vi "subHamamatsu_Snapshot.vi"(7 "Frames to average (1)":i32=1, 8 "Error in":errorcluster, 11 "Value":u32) -> (0 "Error out":errorcluster, 2 "Image":u16[][](graph), 3 "Handle out":u32)   [LabVIEW 2015]
panel:
  # "Take a snapshot and average"
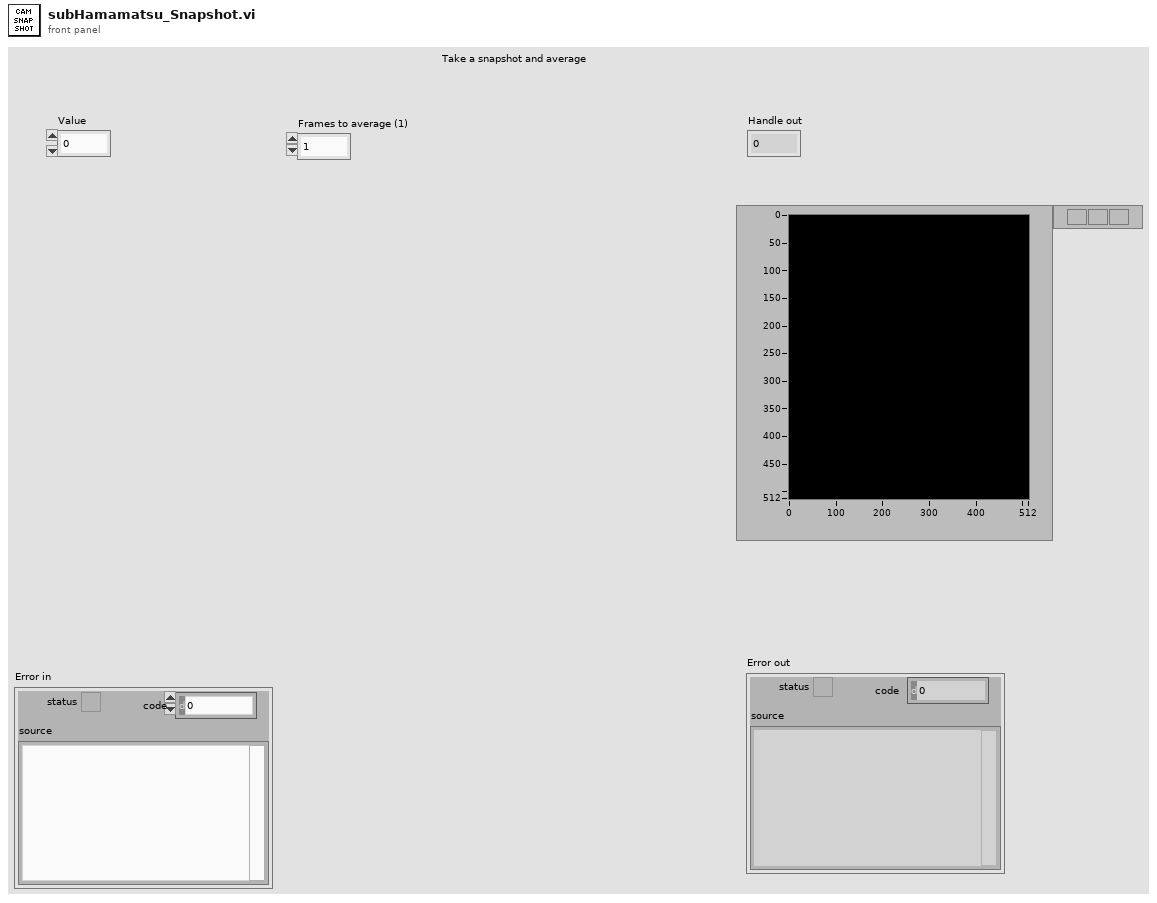
[diagram p1: front panel]
types:
  T1 = cluster{"Value":i32, "Minimum":i32, "Maximum":i32, "Increment":i32}
  T2 = cluster{"width":u32, "height":u32, "datatype":u32}
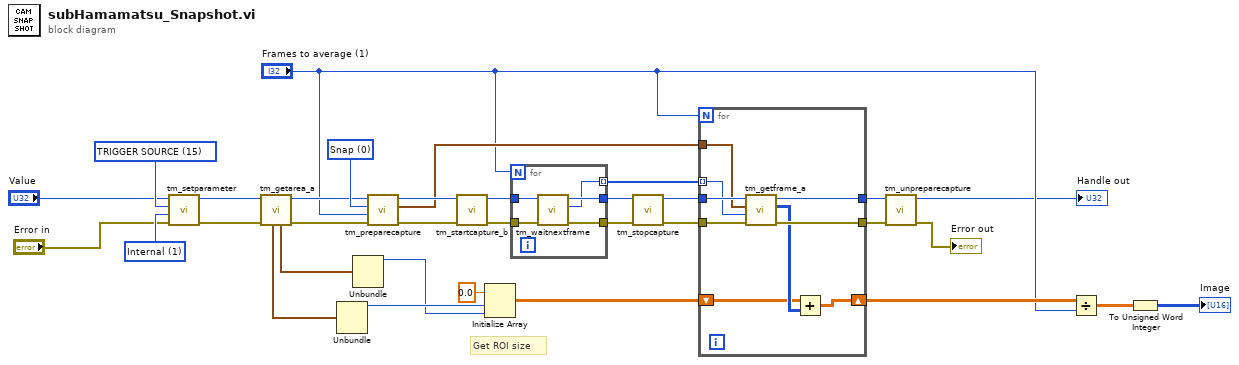
[diagram p0: block diagram]
diagram:
  w32 = 1 items=["Internal"=1, "External"=2, "Software"=3] ("Trigger Source")
  w33 = 15 items=["BINNING"=1, "BITS PER CHANNEL"=2, "ACTIVE VIEW INDEX"=3, "CCD MODE"=4, "SENSOR MODE"=5, "READOUT MODE"=6, "EXPOSURE TIME"=7, "CONTRAST GAIN"=8, "CONTRAST OFFSET"=9, "LIGHT MODE"=10, "SENSITIVITY"=11, "WHITE BALANCE"=12, "PHOTON IMAGING MODE"=13, "HIGH DYNAMIC RANGE MODE"=14, "TRIGGER SOURCE"=15, "TRIGGER ACTIVE"=16, "TRIGGER MODE"=17, "TRIGGER POLARITY"=18, "TRIGGER GLOBAL EXPOSURE"=19, "FIRST TRIGGER BEHAVIOR"=20, "TRIGGER TIMES"=21, "OUTPUT TRIGGER POLARITY"=22, "OUTPUT TRIGGER DELAY"=23, "OUTPUT TRIGGER PERIOD"=24, "TEMPERATURE"=25, "TEMPERATURE TARGET"=26, "SENSOR COOLER FAN"=27, "MECHANICAL SHUTTER"=28, "BACK FOCUS POSITION"=29, "FRAMEBUNDLE MODE"=30, "FRAMEBUNDLE NUMBER"=31, "LINEBUNDLE HEIGHT"=32, "TRIGGER CONNECTOR"=33, "IMAGE PIXEL TYPE"=34] ("Parameter")
  w31 = 0 items=["Snap", "Sequence"] ("Capture mode")
  # "Get ROI size"
  n1 = call "tm_setparameter.vi"("error in (no error)"="Error in", "Value in"=w32, "Parameter"=w33, "Handle in"="Value") -> ("error out"=w3:errorcluster, "Handle out"=w4:u32)  [unwired: 6 in]
  n2 = call "tm_getarea_a.vi"("error in (no error)"=w3, "Handle in"=w4) -> ("error out"=w6:errorcluster, "Handle out"=w7:u32, "H Width"=w11:T1, "V Width"=w12:T1)  [unwired: 4 in, 2 out]
  n3 = Unbundle(w12) -> ("Value"=w10:i32)  [unwired: 3 out]
  n4 = Unbundle(w11) -> ("Value"=w9:i32)  [unwired: 3 out]
  n5 = call "tm_preparecapture.vi"("error in (no error)"=w6, "Frames"="Frames to average (1)", "Capture mode"=w31, "Handle in"=w7) -> ("error out"=w22:errorcluster, "Buffer"=w20:T2, "Handle out"=w21:u32)  [unwired: 4 in, 1 out]
  n6 = call "tm_startcapture_b.vi"("error in (no error)"=w22, "Handle in"=w21) -> ("error out"=w25:errorcluster, "Handle out"=w24:u32)  [unwired: 8 in]
  n7 = Initialize Array(0.0 ("element"), w10, w9) -> (w8:dbl[][])
  n8 = for {
    N: "Frames to average (1)" -> [_]
    tunnel: w24 -> [w38]
    tunnel: w25 -> [w37]
    tunnel: [w36] -> w27
    tunnel: [w35] -> w26
    tunnel: [w34] -> w28 mode=indexing
    n9 = call "tm_waitnextframe.vi"("error in (no error)"=w37, "Handle in"=w38) -> ("error out"=w36:errorcluster, "Frame Index"=w34:i32, "Handle out"=w35:u32)  [unwired: 6 in, 1 out]
  }
  n10 = call "tm_stopcapture.vi"("error in (no error)"=w27, "Handle in"=w26) -> ("error out"=w14:errorcluster, "Handle out"=w15:u32)  [unwired: 8 in]
  n11 = for {
    N: "Frames to average (1)" -> [_]
    tunnel: w15 -> [w47]
    tunnel: w14 -> [w46]
    tunnel: w20 -> [w45]
    tunnel: [w44] -> w30
    tunnel: w28 -> [w43] mode=indexing
    shift-right: [w40] -> w18
    shift-left: w8 -> [w41]
    tunnel: [w39] -> w29
    n12 = call "tm_getframe_a.vi"("error in (no error)"=w46, "Frame Index"=w43, "Buffer"=w45, "Handle in"=w47) -> ("error out"=w44:errorcluster, "Data 16"=w42:u16[][], "Handle out"=w39:u32)  [unwired: 4 in, 1 out]
    n13 = Add(x=w41, y=w42) -> (x+y=w40:dbl[][])
  }
  n14 = call "tm_unpreparecapture.vi"("error in (no error)"=w30, "Handle in"=w29) -> ("error out"=→"Error out":errorcluster, "Handle out"=→"Handle out":u32)  [unwired: 8 in]
  n15 = Divide(x=w18, y="Frames to average (1)") -> (x/y=w19:dbl[][])
  n16 = To Unsigned Word Integer(number=w19) -> (unsigned 16bit integer=→"Image":u16[][])
